vi "CalcJointTorque.vi"(8 "error in (no error)":errorcluster, 10 "CAlexVersion":T1, 11 "Path":path) -> (0 "error out":errorcluster, 1 "AverageTorque":T2, 2 "Torques":T4, 3 "Torque Errors":T3, 5 "ExtraWeight(kg)":cluster{"Thigh":dbl, "Shank":dbl}, 7 "match substring":string)   [LabVIEW 2016]
uses:
  Classes/CAlex2/TypeDef/CAlexVersion.ctl
  CAlex2-Data/CAlex2_Data.lvclass
  <vilib>/Analysis/5stat.llb/RMS (DBL).vi
  <vilib>/Analysis/NI_AALPro.lvlib
  Classes/CAlex2/CAlex2.lvclass
panel:
  out "Planned Torque 4":dbl[][](graph)
  out "Planned Torque 3":dbl[][](graph)
  out "PID Error":dbl[](array[numeric])
  out "Planning Error":dbl[](array[numeric])
  out "All Error":dbl[](array[numeric])
  out "Planed Torque":dbl[][](graph)
  out "Desired Torque":dbl[][](graph)
  out "Acutal Torque":dbl[][](graph)
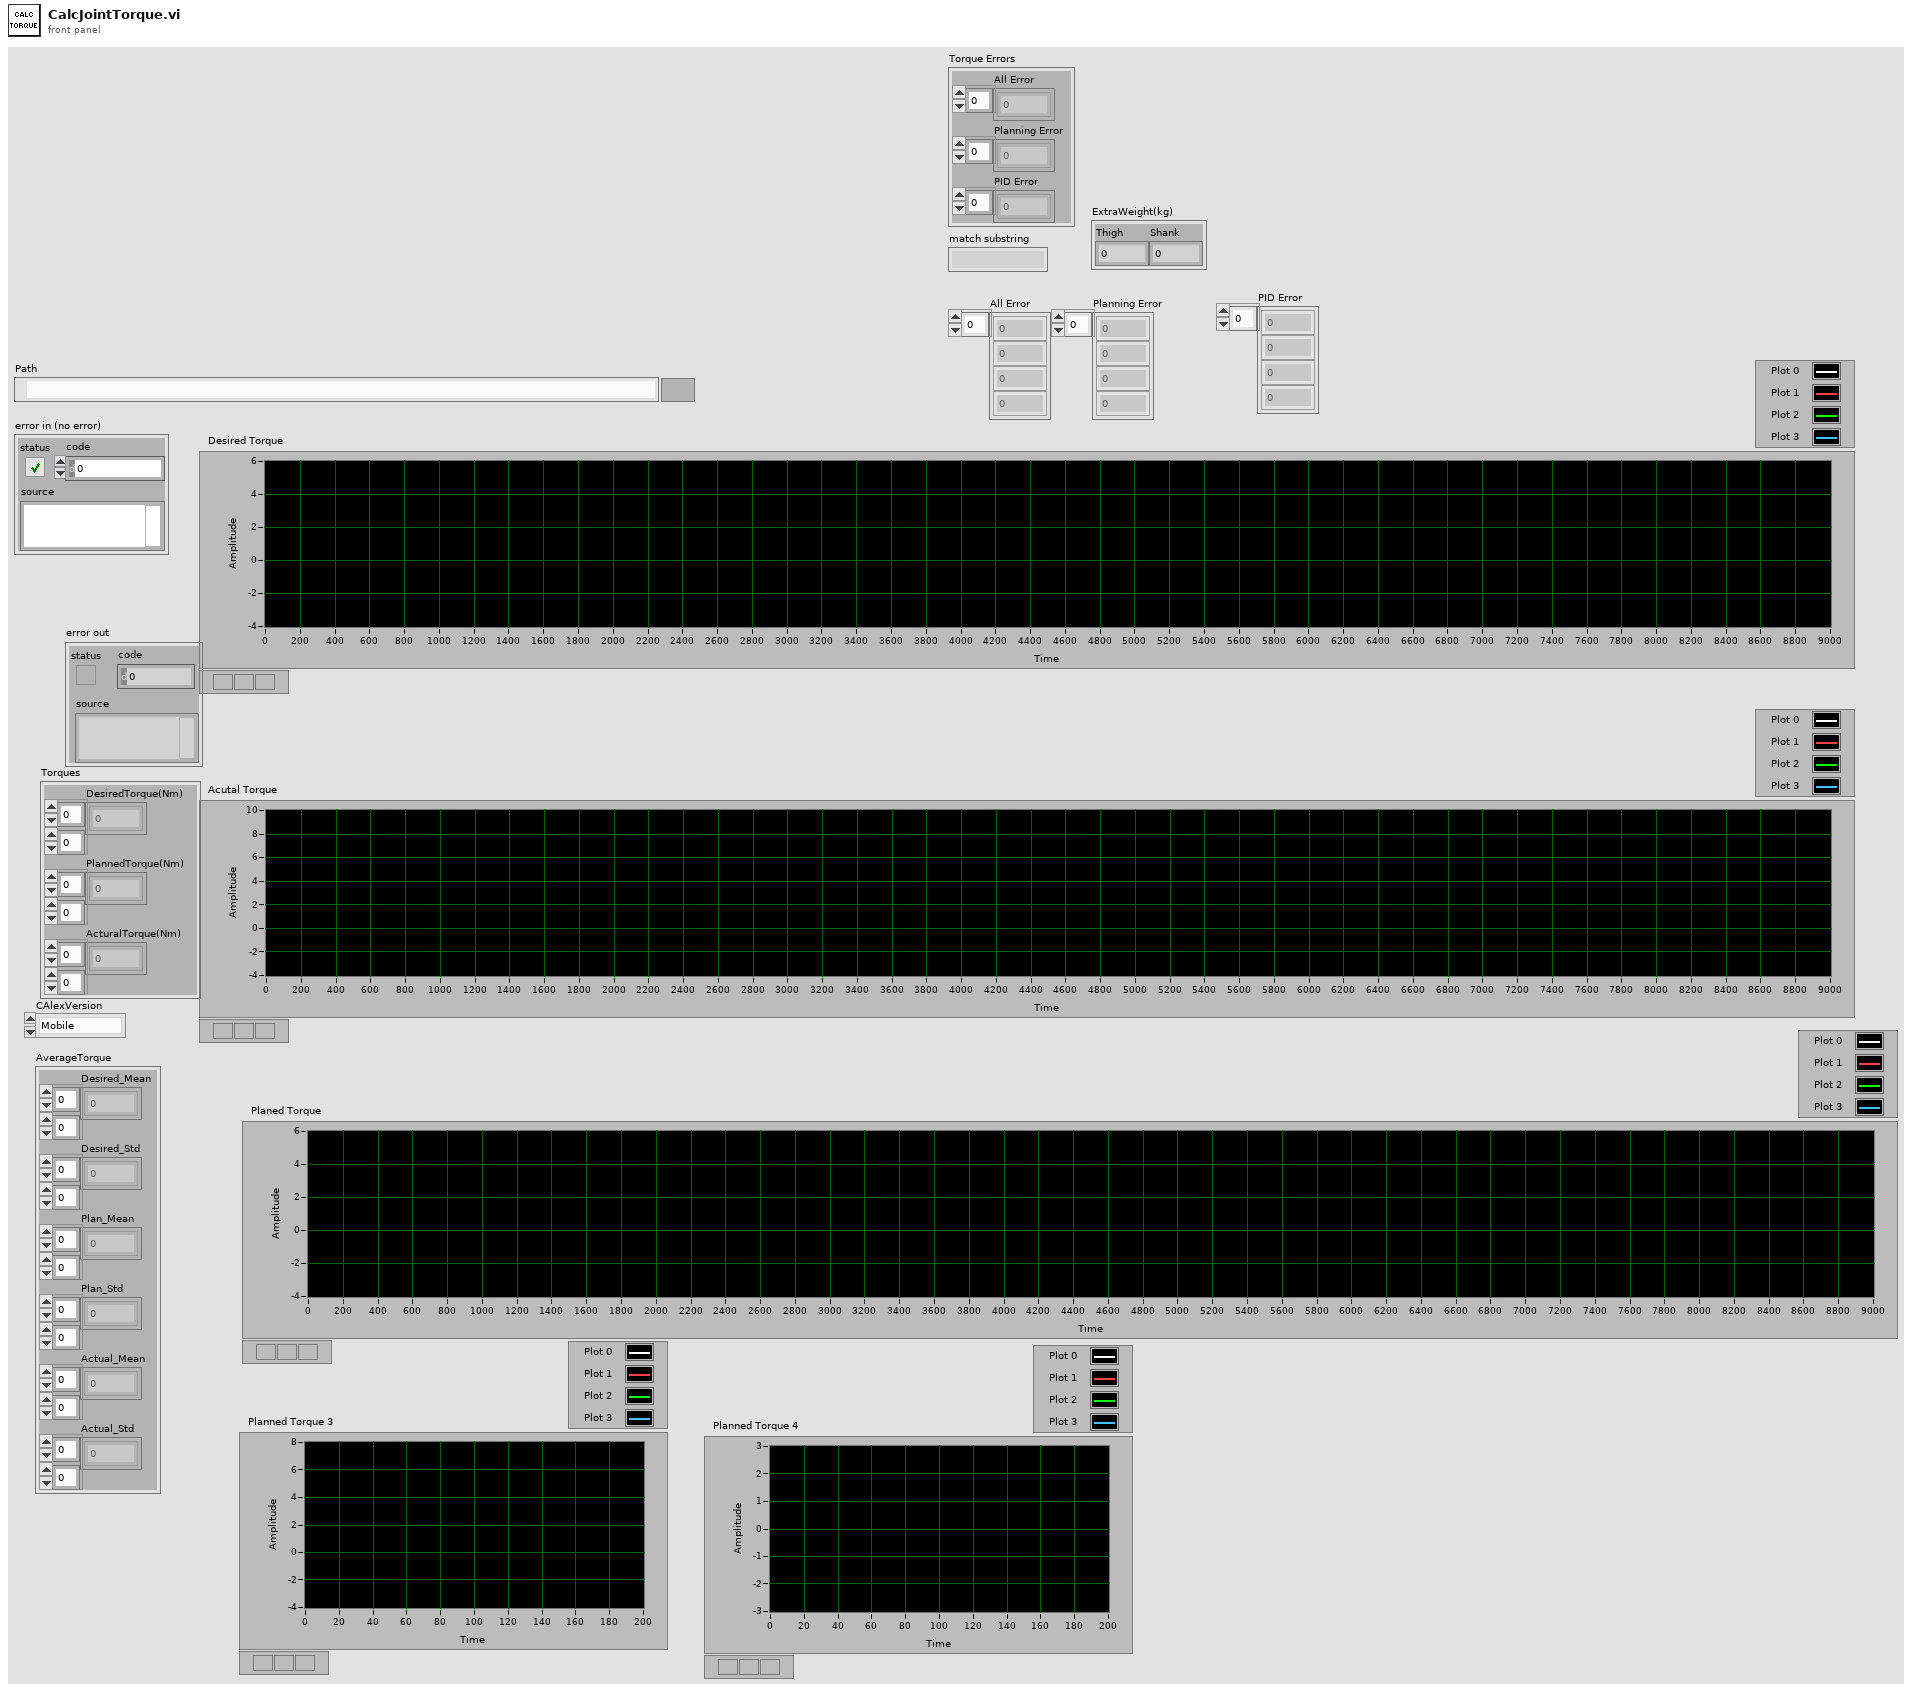
[diagram p1: front panel]
types:
  T1 = typedef "CAlex2.lvclass/CAlexVersion.ctl" = enum16{"Mobile", "Treadmill"}
  T2 = cluster{"Desired_Mean":dbl[][], "Desired_Std":dbl[][], "Plan_Mean":dbl[][], "Plan_Std":dbl[][], "Actual_Mean":dbl[][], "Actual_Std":dbl[][]}
  T3 = cluster{"All Error":dbl[], "Planning Error":dbl[], "PID Error":dbl[]}
  T4 = cluster{"DesiredTorque(Nm)":dbl[][], "PlannedTorque(Nm)":dbl[][], "ActuralTorque(Nm)":dbl[][]}
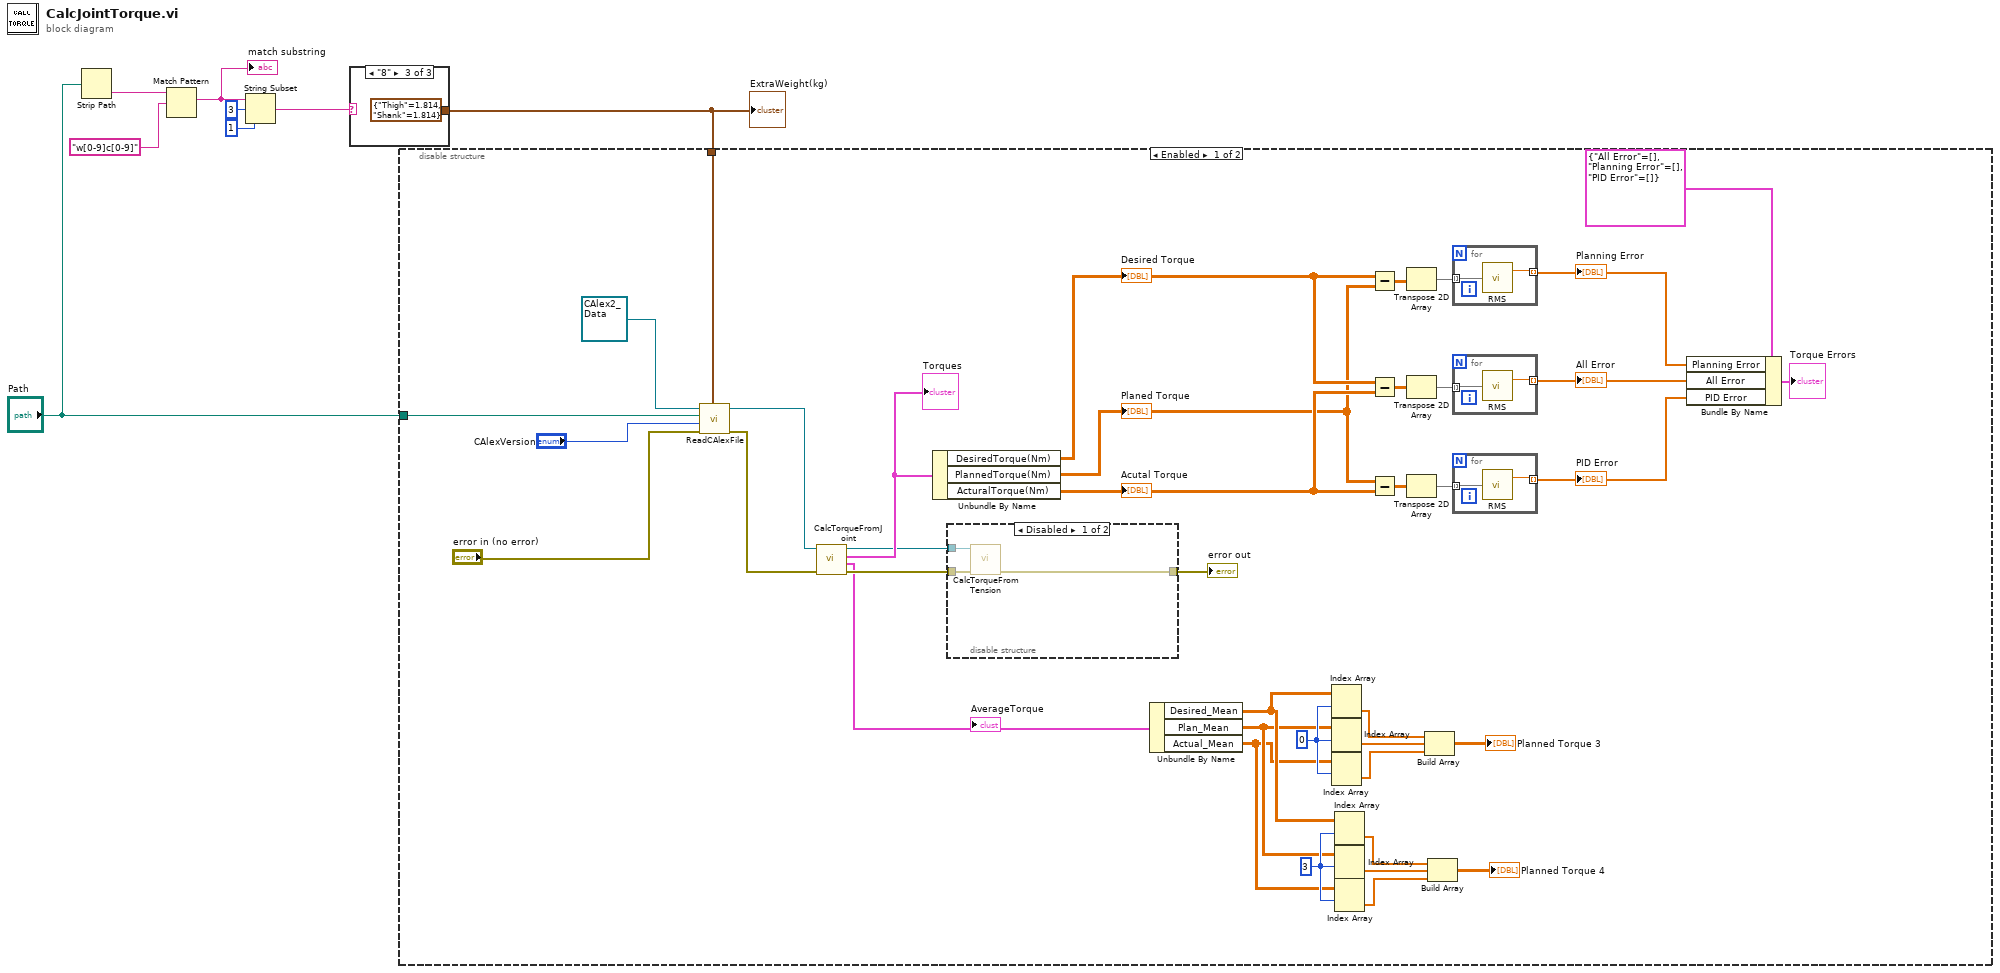
[diagram p0: block diagram]
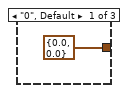
[diagram p4: hidden frame]
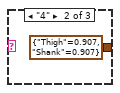
[diagram p5: hidden frame]
diagram:
  n1 = Strip Path(path="Path") -> (name=w7:string)  [unwired: 1 out]
  n2 = Match Pattern(string=w7, regular expression="w[0-9]c[0-9]") -> (match substring=w5:string)  [unwired: 1 in, 3 out]
  "match substring" <- w5
  n3 = String Subset(string=w5, offset (0)=3, length (rest)=1 ("length (rest)")) -> (substring=w2:string)
  n4 = case shown="\"8\"" w2 {
    tunnel: [cluster{"Thigh":dbl, "Shank":dbl} {"Thigh"=0.0, "Shank"=0.0} ("ExtraWeight(kg)") cluster{"Thigh":dbl, "Shank":dbl} {"Thigh"=0.907, "Shank"=0.907} ("ExtraWeight(kg)") cluster{"Thigh":dbl, "Shank":dbl} {"Thigh"=1.814, "Shank"=1.814} ("ExtraWeight(kg)")] -> w1
    frame "0", Default {
    }
    frame "4" {
    }
    frame "8" {
    }
  }
  "ExtraWeight(kg)" <- w1
  n5 = disable-structure shown="Enabled" {
    disable-tunnel: "Path" -> [w34 _]
    disable-tunnel: w1 -> [w32 _]
    frame Enabled {
      w20 = 3 ("index (row)")
      w21 = 0 ("index (row)")
      n6 = call "ReadCAlexFile.vi"("ExtraWeight(kg)"=w32, "error in (no error)"="error in (no error)", "CAlexVersion"="CAlexVersion", "ExpData File Path"=w34, "CAlexData2"=refnum<class "CAlex2_Data.lvclass"> refnum) -> ("error out"=w47:errorcluster, "CAlexData 2"=w48:refnum<class "CAlex2_Data.lvclass">)  [unwired: 5 in]
      n7 = call "CalcTorqueFromJoint.vi"("error in (no error)"=w47, "CAlexData2 in"=w48) -> ("error out"=w44:errorcluster, "AverageTorque"=w26:T2, "Torques"=w46:T4, "CarexMData out"=w45:refnum<class "CAlex2_Data.lvclass">)  [unwired: 5 in, 1 out]
      "Torques" <- w46
      "AverageTorque" <- w26
      n8 = Unbundle By Name(w46) -> ("DesiredTorque(Nm)"=w43:dbl[][], "PlannedTorque(Nm)"=w39:dbl[][], "ActuralTorque(Nm)"=w40:dbl[][])
      "Acutal Torque" <- w40
      "Desired Torque" <- w43
      "Planed Torque" <- w39
      n9 = disable-structure shown="Disabled" {
        disable-tunnel: w45 -> [w55 _]
        disable-tunnel: w44 -> [w54 w56]
        disable-tunnel: [w51 w56] -> w33
        frame Disabled {
          n10 = call "CalcTorqueFromTension.vi"("error in (no error)"=w54, "CAlexData2 in"=w55) -> ("error out"=w51:errorcluster, "Joint Torque Actual"=w52:dbl[][], "Joint Torque Desired"=w53:dbl[][])  [unwired: 4 in, 3 out]
        }
        frame Enabled {
        }
      }
      "error out" <- w33
      n11 = Unbundle By Name(w26) -> ("Desired_Mean"=w15:dbl[][], "Plan_Mean"=w14:dbl[][], "Actual_Mean"=w13:dbl[][])
      n12 = Index Array(array=w15, index (row)=w21) -> (element=w23:dbl[])  [unwired: 1 in]
      n13 = Index Array(array=w14, index (row)=w21) -> (element=w24:dbl[])  [unwired: 1 in]
      n14 = Index Array(array=w13, index (row)=w21) -> (element=w25:dbl[])  [unwired: 1 in]
      n15 = Index Array(array=w15, index (row)=w20) -> (element=w18:dbl[])  [unwired: 1 in]
      n16 = Index Array(array=w14, index (row)=w20) -> (element=w17:dbl[])  [unwired: 1 in]
      n17 = Index Array(array=w13, index (row)=w20) -> (element=w16:dbl[])  [unwired: 1 in]
      n18 = Subtract(x=w43, y=w39) -> (x-y=w42:dbl[][])
      n19 = Subtract(x=w43, y=w40) -> (x-y=w37:dbl[][])
      n20 = Subtract(x=w39, y=w40) -> (x-y=w35:dbl[][])
      n21 = Transpose 2D Array(2D array=w42) -> (transposed array=w41:dbl[][])
      n22 = Transpose 2D Array(2D array=w37) -> (transposed array=w38:dbl[][])
      n23 = Transpose 2D Array(2D array=w35) -> (transposed array=w36:dbl[][])
      n24 = Build Array(w23, w24, w25) -> (→"Planned Torque 3":dbl[][])
      n25 = Build Array(w18, w17, w16) -> (→"Planned Torque 4":dbl[][])
      n26 = for {
        tunnel: w41 -> [w62] mode=indexing
        tunnel: [w61] -> w31 mode=indexing
        n27 = call-poly <vilib>:"RMS.vi"("X"=w62) -> ("rms value"=w61:dbl)  [unwired: 1 out]
      }
      "Planning Error" <- w31
      n28 = for {
        tunnel: w38 -> [w60] mode=indexing
        tunnel: [w59] -> w30 mode=indexing
        n29 = call-poly <vilib>:"RMS.vi"("X"=w60) -> ("rms value"=w59:dbl)  [unwired: 1 out]
      }
      "All Error" <- w30
      n30 = for {
        tunnel: w36 -> [w58] mode=indexing
        tunnel: [w57] -> w29 mode=indexing
        n31 = call-poly <vilib>:"RMS.vi"("X"=w58) -> ("rms value"=w57:dbl)  [unwired: 1 out]
      }
      "PID Error" <- w29
      n32 = Bundle By Name(cluster=T3 {"All Error"=[], "Planning Error"=[], "PID Error"=[]}, "Planning Error"=w31, "All Error"=w30, "PID Error"=w29) -> (→"Torque Errors":T3)
    }
    frame Disabled {
    }
  }
